vi "DSG Generate Waveform.vi"(6 "hardware commands sync queue":T2, 7 "measurement configuration":T1={"Number of channels to measure"=0, "Full scale range"=10.0, "Analog source input channels"=[], "Analog source resource names"=[], "Frequency"=1000.0, "Amplitude"=-1.0, "Digital capture resource name"="", "Digital capture sample rate"=800000.0, "Digital capture samples"=800000}, 8 "error in":errorcluster, 10 "DAQmx product name":string, 11 "DSG task in":refnum<k21>) -> (0 "error out":errorcluster, 3 "DSG task out":refnum<k21>)   [LabVIEW 2021, in "adc_acMultiChannelMeasurement.lvlib"]
uses:
  adc_acMultiChannelMeasurement.lvlib
  shared/subVIs/controls/HW Sync Commands Queue Ref.ctl
  shared/subVIs/controls/HW Sync Commands.ctl
  Measurement Configuration.ctl
  <vilib>/addons/_NISVFA/_Generation/Signal Generation/SV Signal/sv_System Timing Model.ctl
  <vilib>/DAQmx/write.llb/DAQmx Write (Analog 1D Wfm NChan NSamp).vi
  <vilib>/addons/_NISVFA/_Generation/Signal Generation/SV Sinusoid/SV Sinusoid.lvclass
  C:/Program Files/National Instruments/LabVIEW 2021/vi.lib/addons/_NISVFA/_Generation/Signal Generation/SV Signal/SV Signal.lvclass
  <vilib>/addons/_NISVFA/_Generation/Signal Generation/SV Sinusoid/Configure Sine.vi
  <vilib>/addons/_NISVFA/_Generation/Signal Generation/SV Signal/Write Sample Rate.vi
  <vilib>/addons/_NISVFA/_Generation/Signal Generation/SV Signal/Write System Timing Model.vi
  <vilib>/addons/_NISVFA/_Generation/Signal Generation/SV Signal/Write Ramp Parameters.vi
  <vilib>/DAQmx/miscellaneous.llb/DAQmx Fill In Error Info.vi
  <resource>/objmgr/daqmx.rc
  <vilib>/addons/_NISVFA/_Generation/Signal Generation/SV Signal/SV Signal.lvclass
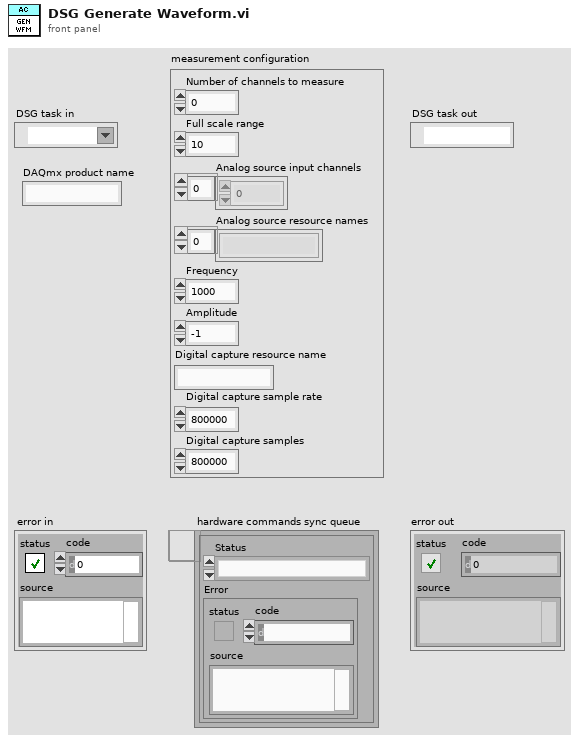
[diagram p1: front panel]
types:
  T1 = typedef "adc_acMultiChannelMeasurement.lvlib/Measurement Configuration.ctl" = cluster{"Number of channels to measure":i32, "Full scale range":dbl, "Analog source input channels":i32[], "Analog source resource names":string[], "Frequency":dbl, "Amplitude":dbl, "Digital capture resource name":string, "Digital capture sample rate":dbl, "Digital capture samples":u32}
  T2 = typedef "HW Sync Commands Queue Ref.ctl" = refnum<queue>
  T3 = enum16{"NoAction", "GenerationStarted", "AcquisitionCompleted", "GenerationErrored"}
  T4 = cluster{"profile":enum16{"Linear", "Half cosine"}, "durations [s]":cluster{"ramp-up":dbl, "transition":dbl, "ramp-down":dbl}}
  T5 = typedef "HW Sync Commands.ctl" = enum16{"NoAction", "GenerationStarted", "AcquisitionCompleted", "GenerationErrored"}
  T6 = cluster{"element":enum16{"NoAction", "GenerationStarted", "AcquisitionCompleted", "GenerationErrored"}, "error out":errorcluster}
  T7 = typedef "SV Signal.lvclass/sv_System Timing Model.ctl" = i64
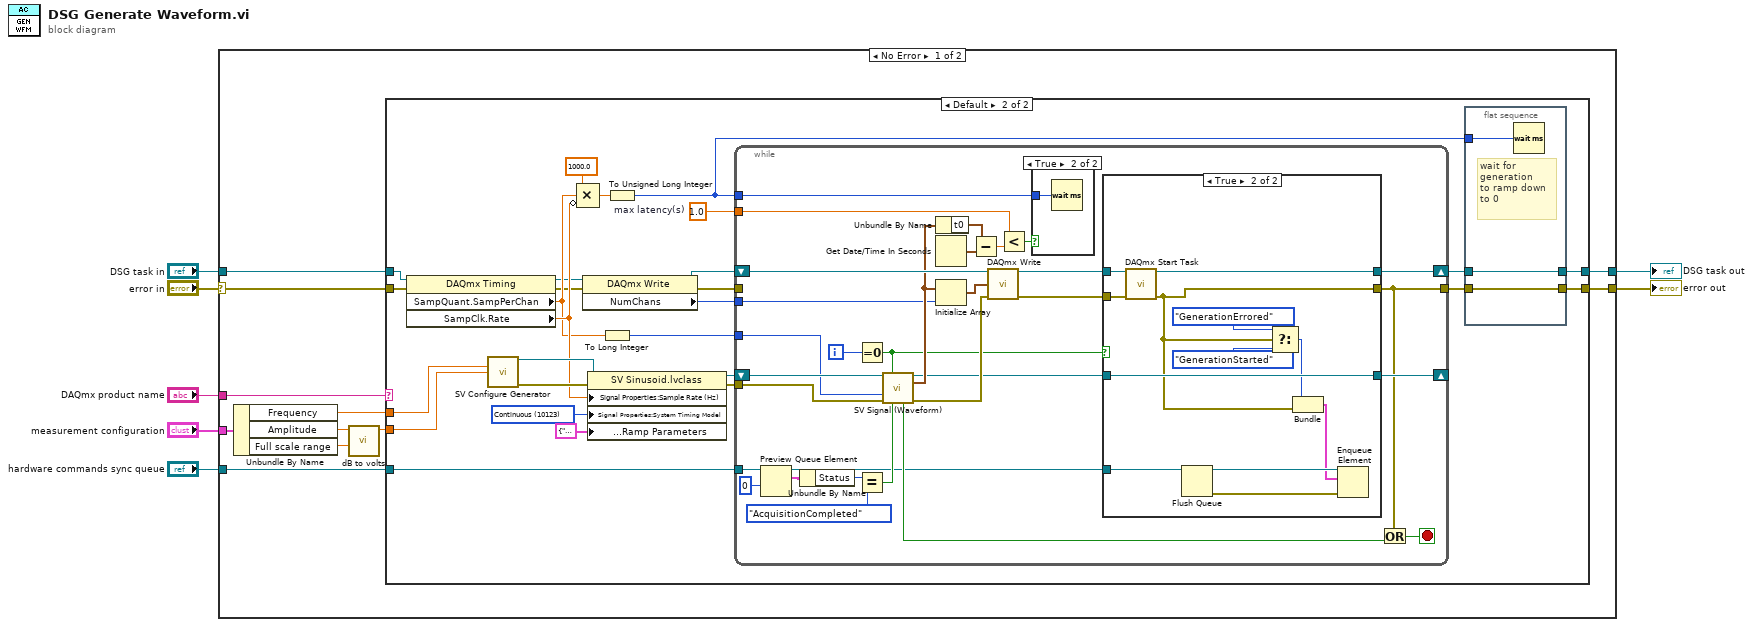
[diagram p0: block diagram]
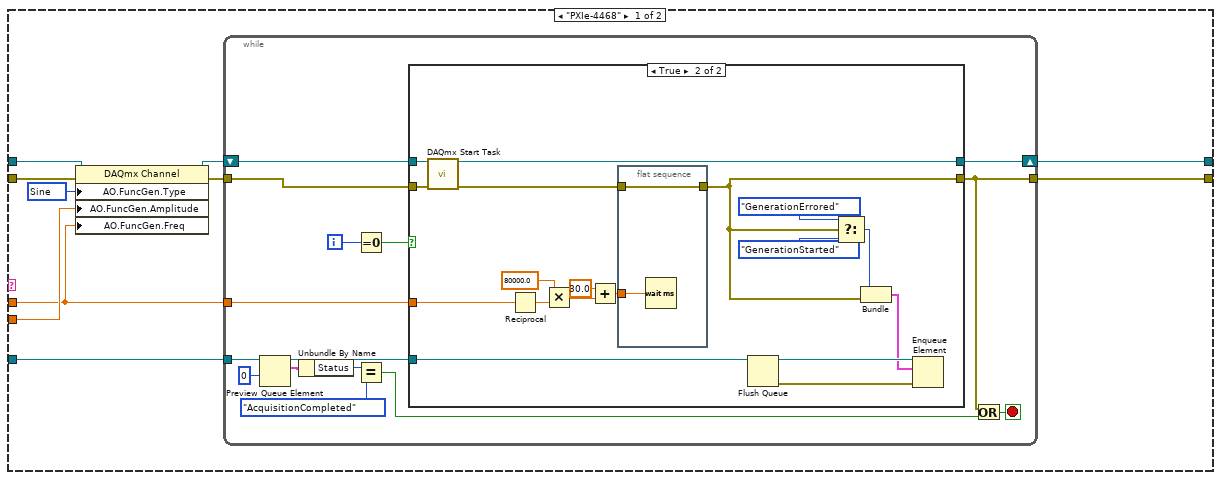
[diagram p2: hidden frame]
diagram:
  n1 = case shown="No Error" "error in" {
    selector: "error in" -> [w18 w144]
    tunnel: [w17 w143] -> w6
    tunnel: [w16 w144] -> w5
    tunnel: "DSG task in" -> [w10 w143]
    tunnel: "hardware commands sync queue" -> [w15 _]
    tunnel: "measurement configuration" -> [w14 _]
    tunnel: "DAQmx product name" -> [w9 _]
    frame No Error {
      n2 = Unbundle By Name(w14) -> ("Frequency"=w12:dbl, "Amplitude"=w13:dbl, "Full scale range"=w8:dbl)
      n3 = call "dB to volts.vi"("Full scale range"=w8, "Voltage(dB)"=w13) -> ("Voltage(volts)"=w11:dbl)  [unwired: 9 in]
      n4 = case shown="Default" w9 {
        tunnel: w18 -> [w22 w92]
        tunnel: w10 -> [w24 w71]
        tunnel: [w27 w78] -> w17
        tunnel: [w26 w77] -> w16
        tunnel: w15 -> [w28 w75]
        tunnel: w12 -> [w19 w73]
        tunnel: w11 -> [w20 w72]
        frame "PXIe-4468" {
          w21 = 14751 items=["Sine"=14751, "Triangle"=14752, "Square"=14753, "Sawtooth"=14754] ("AO.FuncGen.Type")
          n5 = property class="DAQmx Channel"(reference=w24, error in=w22, "AO.FuncGen.Type"=w21, "AO.FuncGen.Amplitude"=w20, "AO.FuncGen.Freq"=w19) -> (reference out=w25:refnum<k21>, error out=w23:errorcluster)
          n6 = while {
            tunnel: w23 -> [w42]
            shift-right: [w36] -> w27
            shift-left: w25 -> [w41]
            tunnel: [w29] -> w26
            tunnel: w28 -> [w33]
            tunnel: w19 -> [w30]
            i -> [w43]
            stop <- w40 stop-if-true
            n7 = Preview Queue Element(queue=w33, timeout in ms (-1)=0) -> (queue out=w37:T2, element=w35:cluster{"Status":T5, "Error":errorcluster})  [unwired: 1 in, 2 out]
            n8 = Unbundle By Name(w35) -> ("Status"=w34:T5)
            n9 = Equal To 0?(x=w43) -> (x = 0?=w32:bool)
            n10 = Equal?(x=w34, y=T3."AcquisitionCompleted") -> (x = y?=w31:bool)
            n11 = case shown="True" w32 {
              tunnel: w37 -> [_ w63]
              tunnel: w41 -> [w45 w61]
              tunnel: [w45 w47] -> w36
              tunnel: w42 -> [w44 w60]
              tunnel: [w44 w49] -> w29
              tunnel: w30 -> [_ w46]
              frame False {
              }
              frame True {
                n12 = call <vilib>:"DAQmx Start Task.vi"("task/channels in"=w61, "error in"=w60) -> ("task out"=w47:refnum<k21>, "error out"=w50:errorcluster)  [unwired: 12 in]
                n13 = Reciprocal(x=w46) -> (1/x=w51:dbl)
                n14 = Multiply(x=80000.0, y=w51) -> (x*y=w53:dbl)
                n15 = Add(x=30.0, y=w53) -> (x+y=w48:dbl)
                n16 = flat-sequence {
                  tunnel: w50 -> [w65]
                  tunnel: [w65] -> w49
                  tunnel: w48 -> [w64]
                  frame #0 {
                    n17 = Wait (ms)(milliseconds to wait=w64) -> ()  [unwired: 1 out]
                  }
                }
                n18 = Flush Queue(queue=w63) -> (queue out=w62:T2, error out=w59:errorcluster)  [unwired: 1 in, 1 out]
                n19 = Select(t=T3."GenerationErrored" ("element"), s=w49, f=T3."GenerationStarted" ("element")) -> (s? t:f=w56:T3)
                n20 = Bundle("element"=w56, "error out"=w49) -> (w55:T6)  [unwired: 1 in]
                n21 = Enqueue Element(queue=w62, element=w55, error in (no error)=w59) -> ()  [unwired: 1 in, 3 out]
              }
            }
            n22 = Or(x=w29, y=w31) -> (x .or. y?=w40:bool)
          }
        }
        frame Default {
          w83 = 1.0  # max latency(s)
          w89 = T7 10123 items=["Finite"=10178, "-"=-1, "Continuous"=10123, "-"=-2, "Settled"=110123, "Averaged"=210123, "Discrete Sweep"=310123, "Continuous Sweep"=410123] ("System Timing Model")
          n23 = property class="DAQmx Timing"(reference=w71, error in=w92) -> (reference out=w68:refnum<k21>, error out=w69:errorcluster, "SampQuant.SampPerChan"=w85:dbl, "SampClk.Rate"=w88:dbl)
          n24 = call-poly <vilib>:"SV Configure Generator.vi"("frequency (Hz)"=w73, "amplitude"=w72) -> ("signal configuration"=w90:refnum<class "SV Sinusoid.lvclass">, "error out"=w91:errorcluster)  [unwired: 12 in]
          n25 = Compound Arithmetic op=MULTIPLY(1000.0 ("value"), w85, invert w88) -> (w82:dbl)
          n26 = property class="DAQmx Write"(reference=w68, error in=w69) -> (reference out=w66:refnum<k21>, error out=w67:errorcluster, "NumChans"=w70:u32)
          n27 = property class="SV Sinusoid.lvclass"(reference=w90, error in=w91, "Signal Properties:Sample Rate (Hz)"=w88, "Signal Properties:System Timing Model"=w89, "Signal Properties:Ramps:Ramp Parameters"=T4 {"profile"=enum."Linear", "durations [s]"={"ramp-up"=0.0, "transition"=0.0, "ramp-down"=0.01}} ("Ramp Parameters:All Elements")) -> (reference out=w87:refnum<class "SV Sinusoid.lvclass">, error out=w86:errorcluster)
          n28 = To Long Integer(number=w85) -> (32bit integer=w84:i32)
          n29 = To Unsigned Long Integer(number=w82) -> (unsigned 32bit integer=w76:u32)
          n30 = while {
            shift-right: [w100] -> _
            shift-left: w87 -> [w126]
            tunnel: w86 -> [w123]
            tunnel: w84 -> [w124]
            shift-right: [w103] -> w79
            shift-left: w66 -> [w122]
            tunnel: [w97] -> w80
            tunnel: w83 -> [w113]
            tunnel: w76 -> [w111]
            tunnel: w75 -> [w110]
            tunnel: w70 -> [w96]
            tunnel: w67 -> [_]
            i -> [w125]
            stop <- w118 stop-if-true
            n31 = Preview Queue Element(queue=w110, timeout in ms (-1)=0) -> (queue out=w106:T2, element=w99:cluster{"Status":T5, "Error":errorcluster})  [unwired: 1 in, 2 out]
            n32 = Unbundle By Name(w99) -> ("Status"=w98:T5)
            n33 = Equal To 0?(x=w125) -> (x = 0?=w105:bool)
            n34 = Equal?(x=w98, y=HW_Sync_Commands."AcquisitionCompleted") -> (x = y?=w107:bool)
            n35 = call-dynamic "SV Signal (Waveform).vi"("signal configuration"=w126, "reset"=w105, "samples"=w124, "error in (no error)"=w123, "stop"=w107) -> ("signal configuration"=w101:refnum<class "SV Sinusoid.lvclass">, "output waveform"=w117:waveform(dbl), "done"=w119:bool, "error out"=w120:errorcluster)  [unwired: 5 in, 2 out]
            n36 = Unbundle By Name(w117) -> ("t0"=w116:timestamp)
            n37 = Get Date/Time In Seconds() -> (seconds since 1Jan1904=w115:timestamp)
            n38 = Initialize Array(w117, w96) -> (w121:waveform(dbl)[])
            n39 = Subtract(x=w116, y=w115) -> (x-y=w114:dbl)
            n40 = call-poly <vilib>:"DAQmx Write.vi"("task/channels in"=w122, "data"=w121, "error in"=w120) -> ("task out"=w104:refnum<k21>, "error out"=w102:errorcluster)  [unwired: 10 in, 1 out]
            n41 = Less?(x=w113, y=w114) -> (x < y?=w112:bool)
            n42 = case shown="True" w112 {
              tunnel: w111 -> [_ w142]
              frame False {
              }
              frame True {
                n43 = Wait (ms)(milliseconds to wait=w142) -> ()  [unwired: 1 out]
              }
            }
            n44 = case shown="True" w105 {
              tunnel: w106 -> [_ w141]
              tunnel: w104 -> [w129 w139]
              tunnel: [w129 w138] -> w103
              tunnel: w102 -> [w128 w137]
              tunnel: [w128 w131] -> w97
              tunnel: w101 -> [w127 w133]
              tunnel: [w127 w133] -> w100
              frame False {
              }
              frame True {
                n45 = call <vilib>:"DAQmx Start Task.vi"("task/channels in"=w139, "error in"=w137) -> ("task out"=w138:refnum<k21>, "error out"=w131:errorcluster)  [unwired: 12 in]
                n46 = Flush Queue(queue=w141) -> (queue out=w140:T2, error out=w136:errorcluster)  [unwired: 1 in, 1 out]
                n47 = Select(t=HW_Sync_Commands."GenerationErrored" ("element"), s=w131, f=HW_Sync_Commands."GenerationStarted" ("element")) -> (s? t:f=w132:T5)
                n48 = Bundle("element"=w132, "error out"=w131) -> (w130:cluster{"element":T5, "error out":errorcluster})  [unwired: 1 in]
                n49 = Enqueue Element(queue=w140, element=w130, error in (no error)=w136) -> ()  [unwired: 1 in, 3 out]
              }
            }
            n50 = Or(x=w97, y=w119) -> (x .or. y?=w118:bool)
          }
          n51 = flat-sequence {
            tunnel: w80 -> [w94]
            tunnel: w79 -> [w95]
            tunnel: [w95] -> w78
            tunnel: [w94] -> w77
            tunnel: w76 -> [w93]
            frame #0 {
              # "wait for\ngeneration\nto ramp down\nto 0"
              n52 = Wait (ms)(milliseconds to wait=w93) -> ()  [unwired: 1 out]
            }
          }
        }
      }
    }
    frame Error {
    }
  }
  "DSG task out" <- w6
  "error out" <- w5
